vi "Append Paragraph with Link [ ].vi"(0 "PDF Report":T25(xcontrol), 2 "Text [ ]":T3[](array[typedef]), 11 "error in (no error)":errorcluster, 13 "Image to Add [ ]":T1 {"Scale" format="%#_g %"}) -> (4 "PDF Report duplicate":T25(xcontrol), 15 "error out":errorcluster)   [LabVIEW 2012]
doc: "Appends text with a <B>line feed</B>, at the end, to the PDF report. This text can be <B>aligned</B> (CENTER, JUSTIFY, LEFT, RIGHT) and <B>indented</B>. \n\nIf <B>Font</B> and <B>Pararaph properties</B> are not specified then the <B>Default font</B> and <B>Default paragraph</B> will be use.\n\nThe data type you wire to the <B>Text</B> input determines the polymorphic instance to use.\n\n<B>FRANÇAIS</B>\nAjoute au rapport PDF du texte sous la forme d'un paragraphe terminé avec un \"<B>Line Feed</B>\". Ce texte peut être <B>aligné</B> (CENTER, JUSTIFY, LEFT, RIGHT) et avoir un <B>renfoncement</B> (gauche et droit) pour tout le paragraphe.\n\nSi la police de caractères <B>Font</B> et les propriétés <B>Pararaph properties</B> ne sont pas spécifiés alors la police par défaut <B>Default font</B> et <B>Default paragraph</B> seront utilisées.\n\nLe type de données que vous connectez au terminal <B>Text</B> détermine l'instance polymorphique utilisée.\n\nDeveloped by Jean-Marc Simard\nCopyright © 2010, Exaprom Inc.\nAll rights reserved.\nLicense: BSD\n\nWith iTextSharp 4.1.6 (http://itextsharp.sourceforge.net)\nunder Mozilla Public License Version 1.1\n(http://www.mozilla.org/MPL/MPL-1.1.html)"
uses:
  Controls/PDF Report Xcontrol/PDF Report.xctl
  Controls/Text and hyperlink.ctl
  Controls/Font cluster.ctl
  Controls/Font size.ctl
  Controls/Font color.ctl
  Controls/Paragraphe cluster.ctl
  Controls/Texte alignement.ctl
  Controls/Line spacing.ctl
  Controls/Paragraph indentation.ctl
  Controls/Image to Add [ ].ctl
  Controls/Image Scale.ctl
  C:/Users/MaxCorp/Documents/TopPerm - Base/DLL/itextsharp.dll
  DLL/itextsharp.dll
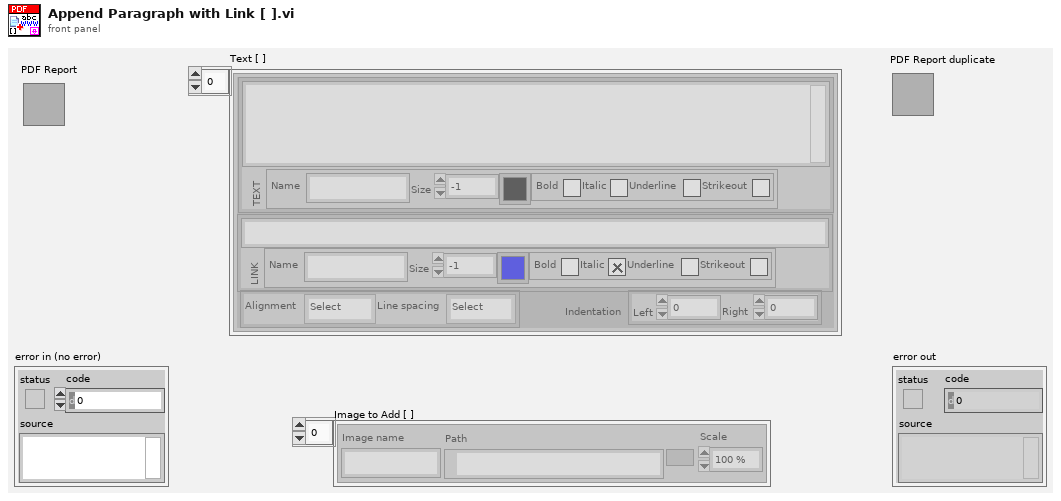
[diagram p1: front panel]
types:
  T1 = typedef "Image to Add [ ].ctl" = cluster{"Image name":string, "Path":path, "Scale":T2}[]
  T2 = typedef "Image Scale.ctl" = sgl
  T3 = typedef "Text and hyperlink.ctl" = cluster{"Text":cluster{"Text":string, "Font":T4}, "Link":cluster{"Hyperlink":string, "Font":T4}, "Paragraphe":T7, "Indentation":T10}
  T4 = typedef "Font cluster.ctl" = cluster{"Name":string, "Size":T5, "Color":T6, "Style":cluster{"Bold":bool, "Italic":bool, "Underline":bool, "Strikeout":bool}}
  T5 = typedef "Font size.ctl" = sgl
  T6 = typedef "Font color.ctl" = u32
  T7 = typedef "Paragraphe cluster.ctl" = cluster{" Aligment":T8, "Line spacing":T9}
  T8 = typedef "Texte alignement.ctl" = enum16{"Select", "CENTER", "JUSTIFY", "LEFT", "RIGHT"}
  T9 = typedef "Line spacing.ctl" = enum16{"Select", "1.0", "1.5", "2.0"}
  T10 = typedef "Paragraph indentation.ctl" = cluster{"Left":sgl, "Right":sgl}
  T11 = typedef "Unit.ctl" = enum16{"inch", "mm"}
  T12 = typedef "Page dimensions.ctl" = cluster{"Start at page":i32, "Orientation":T13, "widht":sgl, "height":sgl, "Margin left":sgl, "Margin right":sgl, "Margin top":sgl, "Margin bottom":sgl}
  T13 = typedef "Page Orientation.ctl" = enum16{"Portrait", "Landscape"}
  T14 = typedef "Image or Table Caption.ctl" = cluster{"Caption":string, "Separator":string, "Position":enum16{"Above", "Below"}}
  T15 = typedef "Header Footer [ ].ctl" = T16[]
  T16 = typedef "Header Footer cluster.ctl" = cluster{"Start page":i32, "Type":T17, "Alignment":T18, "Vertical Alignement":T19, "Image (%)":sgl, "Page #":T20, "Text":string, "Path":string, "Font":T4, "Font refnum":refnum<k24>, "Line":cluster{"Line":T21, "Thickness (points)":sgl, "Colour":T6}}
  T17 = typedef "Header Footer Type.ctl" = enum16{"Select", "Text", "Text + hyperlink", "Page number", "Image", "Image + hyperlink"}
  T18 = typedef "Header footer horiz alignment.ctl" = enum16{"Left", "Center", "Right"}
  T19 = typedef "Cell Vertical alignment.ctl" = enum16{"TOP", "MIDDLE", "BOTTOM"}
  T20 = typedef "Page number.ctl" = cluster{"Text 1":string, "Text 2":string, "Text 3":string}
  T21 = typedef "Header Footer Line.ctl" = enum16{"No line", "Horizontal line"}
  T22 = typedef "Watermark cluster2.ctl" = cluster{"Show? (F)":bool, "Type":enum16{"Image", "Text"}, "Opacity (%)":sgl, "Rotate(°)":sgl, "Position":cluster{"Position":T23, "X":sgl, "Y":sgl}, "Image path":path, "Scaled(%)":sgl, "Image refnum":refnum<k24>, "Text":string, "Font":cluster{"Name":string, "Size":T5, "Color":T6}, "Font refnum":refnum<k24>, "Alignment":T18, "Automatic":bool}
  T23 = typedef "Watermark Position.ctl" = enum16{"Absolute", "Center (page)", "Center (text section)"}
  T24 = typedef "System Fonts.ctl" = cluster{"Font name [ ]":string[], "Font and file names [ ]":cluster{"Font name":string, "File name":string}[]}
  T25 = cluster{"Document":refnum<k24>, "Writer":refnum<k24>, "Default Font":refnum<k24>, "Default Font cluster":T4, "Path":path, "Unit (default = mm)":T11, "Paragraphe cluster":T7, "Pages dimensions [ ]":T12[], "Captions":cluster{"Image":T14, "Image counter":u16, "Table":T14, "Table counter":u16, "Font":T4}, "Header":T15, "Footer":T15, "Watermark ":T22, "Actual VI name":string, "System Fonts":T24}
  T26 = typedef "Image to Add refnum [ ].ctl" = cluster{"Image name":string, "InstanceImage":refnum<k24>}[]
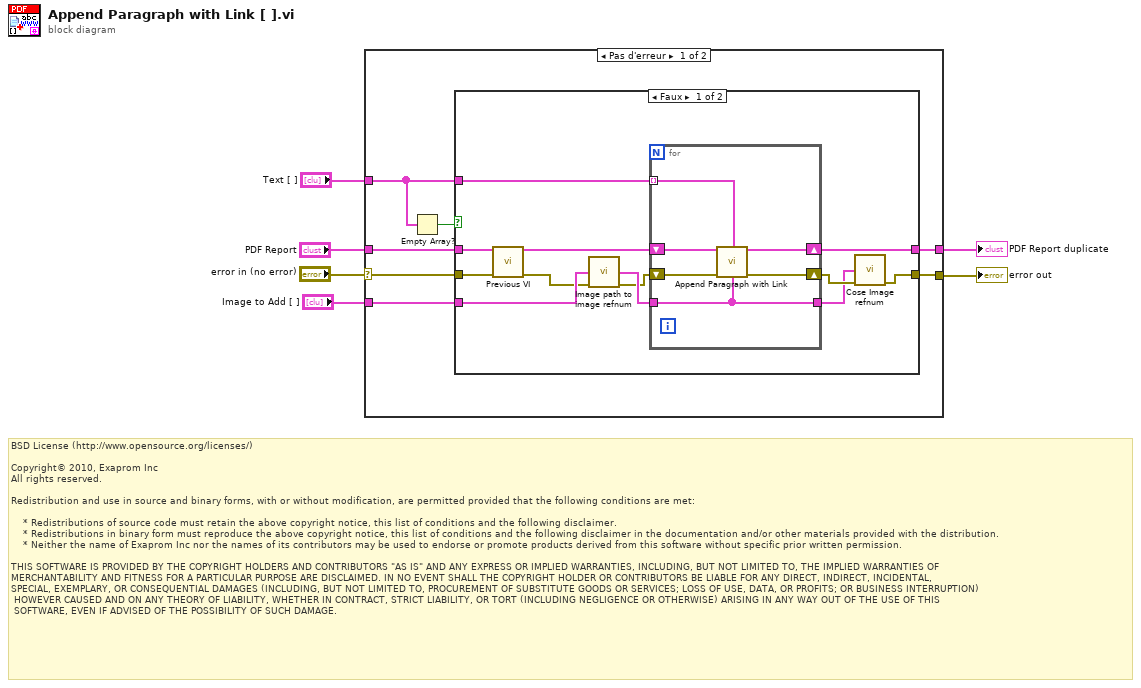
[diagram p0: block diagram]
diagram:
  # "BSD License (http://www.opensource.org/licenses/)\n\nCopyright© 2010, Exaprom Inc\nAll rights reserved.\n\nRedistribution and use in source and binary forms, with or without modification, are permitted provided that the following conditions are met:\n\n    * Redistributions of source code must retain the above copyright notice, this list of conditions and the following disclaimer.\n    * Redistributions in binary form must reproduce the above copyright notice, this list of conditions and the following disclaimer in the documentation and/or other materials provided with the distribution.\n    * Neither the name of Exaprom Inc nor the names of its contributors may be used to endorse or promote products derived from this software without specific prior written permission.\n\nTHIS SOFTWARE IS PROVIDED BY THE COPYRIGHT HOLDERS AND CONTRIBUTORS \"AS IS\" AND ANY EXPRESS OR IMPLIED WARRANTIES, INCLUDING, BUT NOT LIMITED TO, THE IMPLIED WARRANTIES OF \nMERCHANTABILITY AND FITNESS FOR A PARTICULAR PURPOSE ARE DISCLAIMED. IN NO EVENT SHALL THE COPYRIGHT HOLDER OR CONTRIBUTORS BE LIABLE FOR ANY DIRECT, INDIRECT, INCIDENTAL,\nSPECIAL, EXEMPLARY, OR CONSEQUENTIAL DAMAGES (INCLUDING, BUT NOT LIMITED TO, PROCUREMENT OF SUBSTITUTE GOODS OR SERVICES; LOSS OF USE, DATA, OR PROFITS; OR BUSINESS INTERRUPTION)\n HOWEVER CAUSED AND ON ANY THEORY OF LIABILITY, WHETHER IN CONTRACT, STRICT LIABILITY, OR TORT (INCLUDING NEGLIGENCE OR OTHERWISE) ARISING IN ANY WAY OUT OF THE USE OF THIS\n SOFTWARE, EVEN IF ADVISED OF THE POSSIBILITY OF SUCH DAMAGE."
  n1 = case shown="Pas d'erreur" "error in (no error)" {
    selector: "error in (no error)" -> [w12 w35]
    tunnel: [w10 w35] -> w6
    tunnel: "PDF Report" -> [w11 w34]
    tunnel: [w13 w34] -> w3
    tunnel: "Text [ ]" -> [w9 _]
    tunnel: "Image to Add [ ]" -> [w7 _]
    frame No Error {
      n2 = Empty Array?(array=w9) -> (empty?=w8:bool)
      n3 = case shown="Faux" w8 {
        tunnel: [w23 w33] -> w13
        tunnel: w12 -> [w15 w32]
        tunnel: w11 -> [w24 w33]
        tunnel: [w18 w32] -> w10
        tunnel: w9 -> [w25 _]
        tunnel: w7 -> [w22 _]
        frame False {
          n4 = call "Previous VI.vi"("PDF Report IN"=w24, "error in (no error)"=w15) -> ("PDF Report OUT"=w16:T25, "error out"=w14:errorcluster)  [unwired: 12 out]
          n5 = call "Image path to image refnum.vi"("Image to Add [ ]"=w22, "error in (no error)"=w14) -> ("Image to Add refnum [ ]"=w21:T26, "error out"=w20:errorcluster)  [unwired: 12 out]
          n6 = for {
            shift-right: [w29] -> w19
            shift-left: w20 -> [w30]
            shift-right: [w31] -> w23
            shift-left: w16 -> [w28]
            tunnel: w25 -> [w27] mode=indexing
            tunnel: w21 -> [w26]
            tunnel: [w26] -> w17
            n7 = call "Append Paragraph with Link.vi"("PDF Report"=w28, "Text"=w27, "error in (no error)"=w30, "Image to Add refnum [ ]"=w26) -> ("PDF Report duplicate"=w31:T25, "error out"=w29:errorcluster)  [unwired: 10 out]
          }
          n8 = call "Cose Image refnum.vi"("Image to Add refnum [ ]"=w17, "error in (no error)"=w19) -> ("error out"=w18:errorcluster)  [unwired: 13 out]
        }
        frame True {
        }
      }
    }
    frame Error {
    }
  }
  "error out" <- w6
  "PDF Report duplicate" <- w3
